vi "h.NET.SetStaticNetworkSettings.vi"(4 "Gateway":string, 5 "error in":errorcluster, 6 "Netmask":string, 7 "IP Address":string, 8 "Connection ID":refnum<k5>) -> (0 "error out":errorcluster, 2 "Message":string, 3 "Connection ID":refnum<k5>)   [LabVIEW 2016, in "h.Library.lvlib"]
doc: "Sets the static IP configuration for the instrument. This configuration can be set even if the instrument is currently configured by DHCP. Static IP settings take effect when the instrument is switched from dynamic to static configuration. Use the h.SYSTEM.SaveConfig.vi VI to make these settings permanent.\n\n<b>Connection ID</b> - is a network connection refnum that uniquely identifies the TCP connection\n<b>IP Address</b> - sets the static network IP address (dotted quad notation)\n<b>Netmask</b> - optionally sets the static network netmask (dotted quad notation)\n<b>Gateway</b> - optionally sets the static network gateway (dotted quad notation)\n<b>error in</b> - describes error conditions that occur before this node runs. This input provides standard error functionality\n<b>Connection ID out</b> - returns the same value as connection ID\n<b>Message</b> - human readable string reporting the outcome of the executed command\n<b>error out</b> - contains error information. This output provides standard error out functionality."
uses:
  h.Library.lvlib
panel:
  # "Hyperion Set Static Network Settings"
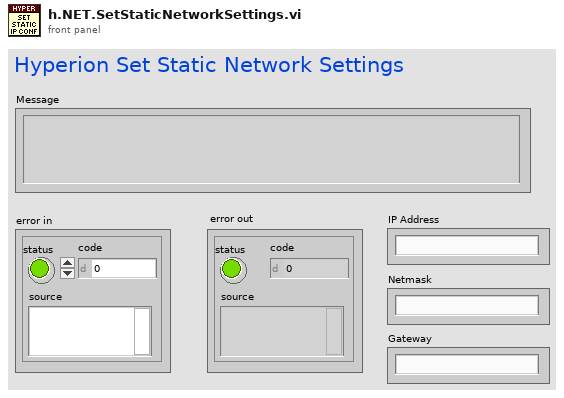
[diagram p1: front panel]
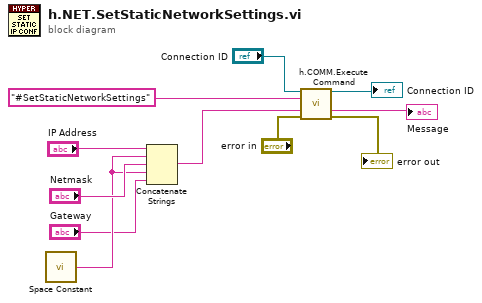
[diagram p0: block diagram]
diagram:
  n1 = call <vilib>:"Space Constant.vi"() -> ("String"=w3:string)
  n2 = Concatenate Strings("IP Address", w3, "Netmask", w3, "Gateway") -> (w1:string)
  n3 = call "h.COMM.Execute Command.vi"("Connection ID"="Connection ID", "Command"="#SetStaticNetworkSettings", "Argument"=w1, "error in"="error in") -> ("Connection ID out"=→"Connection ID":refnum<k5>, "Message"=→"Message":string, "error out"=→"error out":errorcluster)  [unwired: 4 in, 5 out]
